vi "Read Accounts Data.vi"(8 "error in (no error)":errorcluster, 11 "Accounts.txt file path":path) -> (0 "error out":errorcluster, 3 "Accounts info":T1)   [LabVIEW 2020, in "ATM.lvlib"]
doc: "This VI parses the information from the Accounts.txt file selected path and returns the accounts, names, surnames and remaining money."
uses:
  ATM.lvlib
  Account Info -- cluster.ctl
  Accounts Info -- cluster.ctl
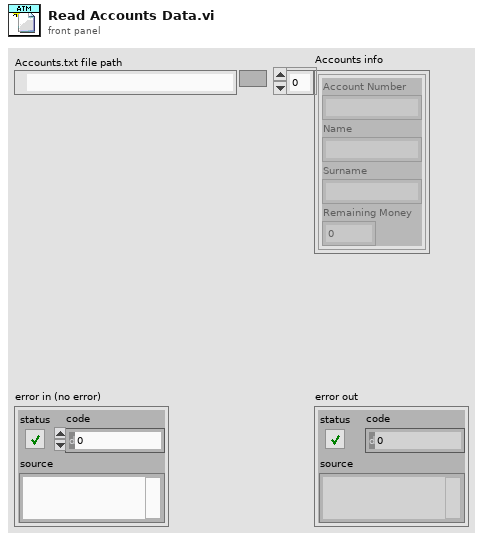
[diagram p1: front panel]
types:
  T1 = typedef "ATM.lvlib/Accounts Info -- cluster.ctl" = T2[]
  T2 = typedef "ATM.lvlib/Account Info -- cluster.ctl" = cluster{"Account Number":string, "Name":string, "Surname":string, "Remaining Money":i32}
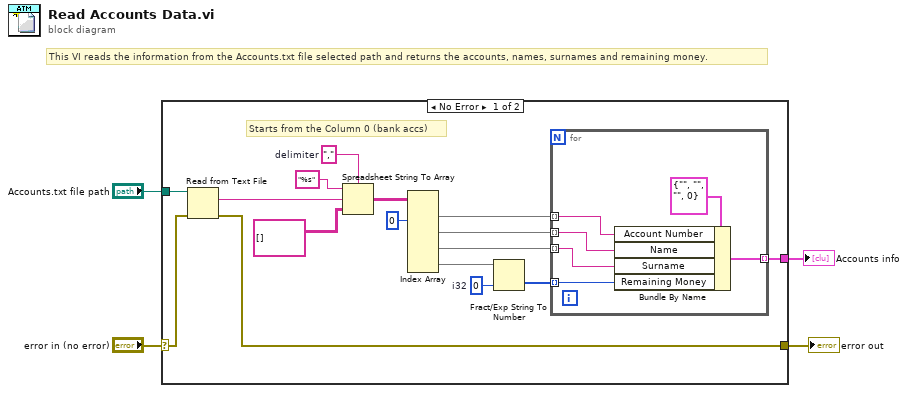
[diagram p0: block diagram]
diagram:
  # "This VI reads the information from the Accounts.txt file selected path and returns the accounts, names, surnames and remaining money."
  n1 = case shown="No Error" "error in (no error)" {
    selector: "error in (no error)" -> [w6 w27]
    tunnel: "Accounts.txt file path" -> [w20 _]
    tunnel: [w5 w27] -> w3
    tunnel: [w10 _] -> w2
    frame No Error {
      w12 = 0  # i32
      w19 = ","  # delimiter
      # "Starts from the Column 0 (bank accs)"
      n2 = Read from Text File(file (use dialog)=w20, error in=w6) -> (text=w18:string, error out=w5:errorcluster)  [unwired: 2 in, 2 out]
      n3 = Spreadsheet String To Array(delimiter (Tab)=w19, format string="%s", spreadsheet string=w18, array type (2D Dbl)=string[][] []) -> (array=w15:string[][])
      n4 = Index Array(array=w15, index (col) #1=0 ("disabled index (col)")) -> (element #1=w7:string[], element #2=w8:string[], element #3=w9:string[], element #4=w13:string[])  [unwired: 7 in]
      n5 = Fract/Exp String To Number(string=w13, default (0 dbl)=w12) -> (number=w11:i32[])  [unwired: 2 in, 1 out]
      n6 = for {
        tunnel: w11 -> [w24] mode=indexing
        tunnel: [w25] -> w10 mode=indexing
        tunnel: w9 -> [w23] mode=indexing
        tunnel: w8 -> [w22] mode=indexing
        tunnel: w7 -> [w21] mode=indexing
        n7 = Bundle By Name(cluster=T2 {"Account Number"="", "Name"="", "Surname"="", "Remaining Money"=0} ("Account Info"), "Account Number"=w21, "Name"=w22, "Surname"=w23, "Remaining Money"=w24) -> (w25:T2)
      }
    }
    frame Error {
    }
  }
  "error out" <- w3
  "Accounts info" <- w2
